vi "Test Config.vi"() -> ()   [LabVIEW 2012]
uses:
  Utilities/FPGA/Controls/FPGAConfig.ctl
  Reusable/PAS/Main/Controls/Laser Modulation.ctl
  <vilib>/Utility/config.llb/Write Key (Boolean).vi
  <vilib>/Utility/config.llb/NI_LVConfig.lvlib
panel:
  out "error out":errorcluster
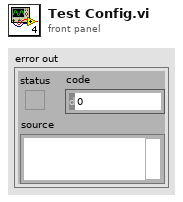
[diagram p1: front panel]
types:
  T1 = typedef "FPGAConfig.ctl" = cluster{"Span":cluster{"ch 1":sgl, "ch 2":sgl, "ch 3":sgl, "ch 4":sgl, "ch 5":sgl}, "mod":cluster{"ch 1":T2, "ch 2":T2, "ch 3":T2, "ch 4":T2, "ch 5":T2}}
  T2 = typedef "Laser Modulation.ctl" = enum8{"Sine", "Square"}
  T3 = typedef "NI_LVConfig.lvlib/Config Data RefNum.ctl" = refnum<k1>
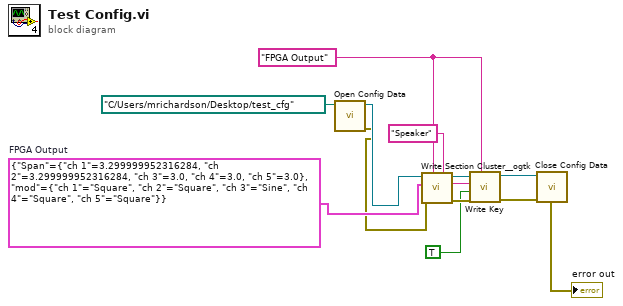
[diagram p0: block diagram]
diagram:
  w3 = "FPGA Output" ("section (optional)")
  w10 = T1 {"Span"={"ch 1"=3.3, "ch 2"=3.3, "ch 3"=3.0, "ch 4"=3.0, "ch 5"=3.0}, "mod"={"ch 1"=enum."Square", "ch 2"=enum."Square", "ch 3"=enum."Sine", "ch 4"=enum."Square", "ch 5"=enum."Square"}}  # FPGA Output
  n1 = call <vilib>:"Open Config Data.vi"("configuration file path"=path "C:/Users/mrichardson/Desktop/test_cfg") -> ("error out"=w9:errorcluster, "refnum"=w11:T3)  [unwired: 8 in, 1 out]
  n2 = call <userlib>:"Write Section Cluster__ogtk.vi"("section (optional)"=w3, "error in (no error)"=w9, "Section Formatted Cluster"=w10, "refnum"=w11) -> ("error out"=w4:errorcluster, "dup refnum"=w5:T3)  [unwired: 6 in]
  n3 = call-poly <vilib>:"Write Key.vi"("section"=w3, "error in (no error)"=w4, "value"=TRUE, "key"="Speaker", "refnum"=w5) -> ("error out"=w7:errorcluster, "refnum out"=w6:T3)  [unwired: 4 in, 1 out]
  n4 = call <vilib>:"Close Config Data.vi"("error in (no error)"=w7, "refnum"=w6) -> ("error out"=→"error out":errorcluster)  [unwired: 8 in, 1 out]
